vi "Init Context Menu.vi"(0 "Menu in":refnum<k9>, 5 "Display State In":T1 caption="State", 7 "Run Mode?":bool) -> (4 "Menu out":refnum<k9>, 8 "Discard":bool)   [LabVIEW 2020, in "PXISlotGP.xctl"]
uses:
  PXISlotGP.xctl
  State.ctl
  PXISlot XControl/Connector Type.ctl
  AOAIRefs.ctl
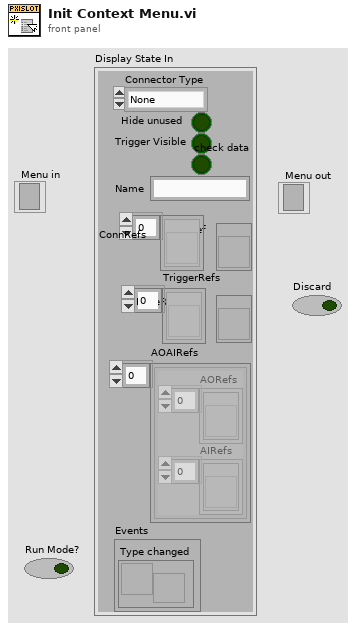
[diagram p1: front panel]
types:
  T1 = typedef "PXISlotGP.xctl/State.ctl" = cluster{"Connector Type":T2, "Hide unused":bool, "Trigger Visible":bool, "TabRef":refnum<vi>, "ConnRefs":refnum<vi>[], "PaneRef":refnum<vi>, "AOAIRefs":T3[], "TriggerRefs":refnum<vi>[], "check data":bool, "Name":string, "Events":cluster{"Type changed":refnum<user-event>}}
  T2 = typedef "Connector Type.ctl" = enum16{"None", "PXI-4461", "BNC-2110", "BNC-2090", "PXIe-4463", "PXIe-4464"}
  T3 = typedef "AOAIRefs.ctl" = cluster{"AORefs":refnum<vi>[], "AIRefs":refnum<vi>[]}
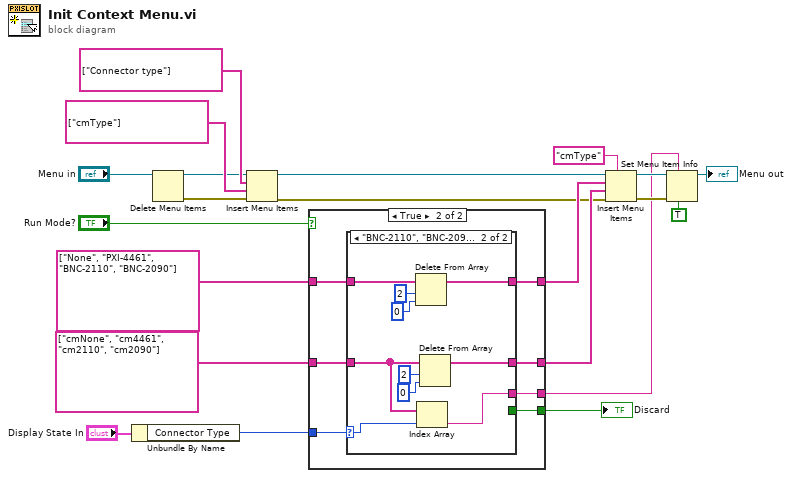
[diagram p0: block diagram]
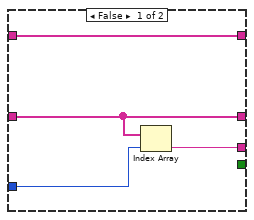
[diagram p2: hidden frame]
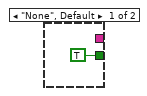
[diagram p3: hidden frame]
diagram:
  n1 = Unbundle By Name("Display State In") -> ("Connector Type"=w15:T2)
  n2 = Delete Menu Items(9:"Menu in") -> (0:w1:errorcluster, 3:w2:refnum<k9>)  [unwired: 3 in]
  n3 = Insert Menu Items(6:w1, 7:string[] ["cmType"] ("item names"), 8:string[] ["Connector type"] ("item names"), 9:w2) -> (0:w4:errorcluster, 3:w5:refnum<k9>)  [unwired: 2 in, 1 out]
  n4 = case shown="True" "Run Mode?" {
    tunnel: string[] ["None", "PXI-4461", "BNC-2110", "BNC-2090"] ("item names") -> [w25 w31]
    tunnel: string[] ["cmNone", "cm4461", "cm2110", "cm2090"] ("item names") -> [w24 w30]
    tunnel: [w25 w29] -> w17
    tunnel: [w24 w28] -> w16
    tunnel: w15 -> [w23 w32]
    tunnel: [_ w27] -> w14
    tunnel: [w22 w26] -> w11
    frame False {
      n5 = Index Array(array=w24, index=w23) -> (element=w22:string)
    }
    frame True {
      n6 = case shown="\"BNC-2110\", \"BNC-2090\"" w32 {
        selector: w32 -> [_ w37]
        tunnel: w31 -> [_ w43]
        tunnel: w30 -> [_ w38]
        tunnel: [_ w41] -> w29
        tunnel: [_ w39] -> w28
        tunnel: [TRUE _] -> w27
        tunnel: [_ w36] -> w26
        frame "None", Default {
        }
        frame "BNC-2110", "BNC-2090" {
          n7 = Delete From Array(array=w43, length=2, index=0) -> (array with subset deleted=w41:string[])  [unwired: 1 out]
          n8 = Index Array(array=w38, index=w37) -> (element=w36:string)
          n9 = Delete From Array(array=w38, length=2, index=0) -> (array with subset deleted=w39:string[])  [unwired: 1 out]
        }
      }
    }
  }
  "Discard" <- w14
  n10 = Insert Menu Items(5:"cmType" ("menu tag"), 6:w4, 7:w16, 8:w17, 9:w5) -> (0:w12:errorcluster, 3:w13:refnum<k9>)  [unwired: 1 in, 1 out]
  n11 = Set Menu Item Info(6:TRUE ("checked"), 7:w11, 8:w12, 11:w13) -> (3:→"Menu out":refnum<k9>)  [unwired: 3 in, 1 out]
